vi "Configure Trigger Level.vi"(7 "Output Function (0: Voltage)":i32(ring) items=["Current", "Voltage"], 8 "error in (no error)":errorcluster, 9 "Trigger Level (0.001)":dbl=0.001, 10 "Channel (1)":string="1", 11 "VISA resource name":refnum<visa-resource-name>) -> (0 "error out":errorcluster, 3 "VISA resource name out":refnum<visa-resource-name>)   [LabVIEW 2020, in "Keysight E36300 Series.lvlib"]
doc: "Configures the trigger level of the specified output channel."
uses:
  Keysight E36300 Series.lvlib
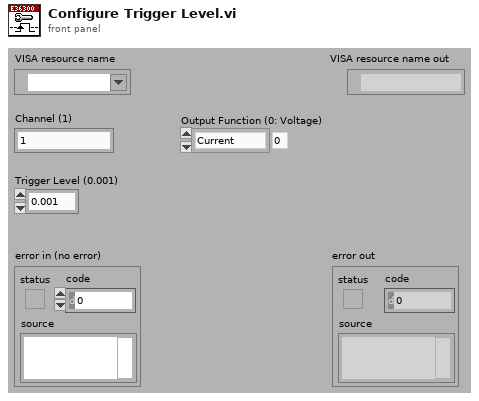
[diagram p1: front panel]
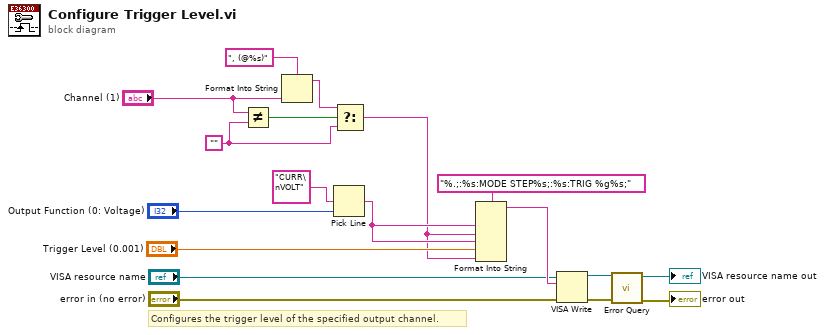
[diagram p0: block diagram]
diagram:
  w1 = ""
  # "Configures the trigger level of the specified output channel."
  n1 = Not Equal?(x="Channel (1)", y=w1) -> (x != y?=w4:bool)
  n2 = Format Into String(format string=", (@%s)", "Channel (1)") -> (resulting string=w5:string)  [unwired: 2 in, 1 out]
  n3 = Pick Line(multi-line string="CURR\nVOLT", line index="Output Function (0: Voltage)") -> (output string=w11:string)  [unwired: 1 in]
  n4 = Select(t=w5, s=w4, f=w1) -> (s? t:f=w2:string)
  n5 = Format Into String(format string="%.;:%s:MODE STEP%s;:%s:TRIG %g%s;", w11, w2, w11, "Trigger Level (0.001)", w2) -> (resulting string=w18:string)  [unwired: 2 in, 1 out]
  n6 = VISA Write(VISA resource name="VISA resource name", write buffer=w18, error in (no error)="error in (no error)") -> (VISA resource name out=w10:refnum<visa-resource-name>, error out=w8:errorcluster)  [unwired: 1 out]
  n7 = call "Error Query.vi"("error in (no error)"=w8, "VISA resource name"=w10) -> ("error out"=→"error out":errorcluster, "VISA resource name out"=→"VISA resource name out":refnum<visa-resource-name>)  [unwired: 6 in, 2 out]
